vi "Manip2.vi"() -> ()   [LabVIEW 2021]
panel:
  out "Kelvin":dbl
  out "Deg F":dbl
  in  "Deg C":dbl
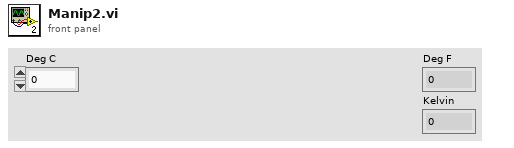
[diagram p1: front panel]
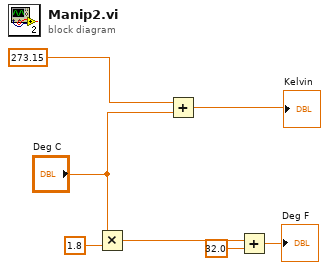
[diagram p0: block diagram]
diagram:
  n1 = Multiply(x="Deg C", y=1.8) -> (x*y=w6:dbl)
  n2 = Add(x=273.15, y="Deg C") -> (x+y=→"Kelvin":dbl)
  n3 = Add(x=w6, y=32.0) -> (x+y=→"Deg F":dbl)
